vi "SVT UFF58 Write Time Waveform (N Ch).vi"(0 "file refnum":refnum<k20>, 1 "ID lines (1-3)":T2[](array[typedef]), 2 "data precision (double-precision:1)":T1=1 items=["single-precision", "double-precision"], 5 "waveforms":waveform(dbl)[](array[waveform]), 11 "error in (no error)":errorcluster) -> (4 "dup file refnum":refnum<k20>, 6 "function refnums":refnum<k20>[](array[refnum]), 15 "error out":errorcluster)   [LabVIEW 2017, in "SoundVib_UFF58.lvlib"]
doc: "Writes data to the UFF58 (universal file format) file specified by the <B>file refnum</B> input. This VI also writes the fields in records 1, 2, and 3, <B>ID lines (1-3)</B>. You can write a single time domain waveform, multiple time domain waveforms, a single real frequency spectrum, multiple real frequency spectra, a single complex frequency spectrum, multiple complex frequency spectra, or generic data to a UFF file. If a frequency spectrum is in decibels, this VI converts the spectrum to linear before writing to the UFF58 file. The default instance, SVT UFF58 Write Time Waveform (1 Ch), writes a single time domain waveform to the file specified by the <B>file refnum</B> input. Wire data to the <B>file refnum</B> input to determine the polymorphic instance to use or manually select the instance."
uses:
  <vilib>/addons/Sound and Vibration/svt_UFF58/SoundVib_UFF58.lvlib
  <vilib>/addons/Sound and Vibration/svt_UFF58/subVIs/sv_IDLines123.ctl
  <vilib>/addons/Sound and Vibration/svt_UFF58/subVIs/sv_UFF58 Data Precision.ctl
  <vilib>/addons/Sound and Vibration/svt_UFF58/subVIs/sv_UFF58 Check Data Valid (Time) (NCh).vi
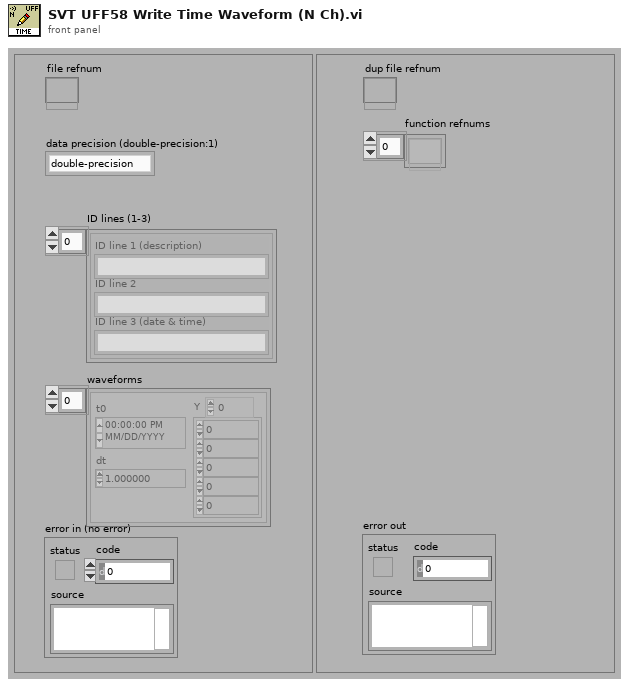
[diagram p1: front panel]
types:
  T1 = typedef "SoundVib_UFF58.lvlib/sv_UFF58 Data Precision.ctl" = u32
  T2 = typedef "SoundVib_UFF58.lvlib/sv_IDLines123.ctl" = cluster{"ID line 1 (description)":string, "ID line 2":string, "ID line 3 (date & time)":string}
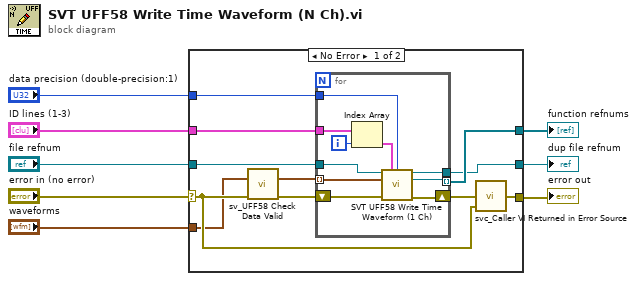
[diagram p0: block diagram]
diagram:
  n1 = case shown="No Error" "error in (no error)" {
    selector: "error in (no error)" -> [w12 w30]
    tunnel: "file refnum" -> [w19 w31]
    tunnel: "ID lines (1-3)" -> [w10 _]
    tunnel: "waveforms" -> [w11 _]
    tunnel: [w18 _] -> w5
    tunnel: [w13 w30] -> w4
    tunnel: [w17 w31] -> w3
    tunnel: "data precision (double-precision:1)" -> [w9 _]
    frame No Error {
      n2 = call-poly <vilib>:"sv_UFF58 Check Data Valid.vi"("waveforms"=w11, "error in (no error)"=w12) -> ("dup waveforms"=w16:waveform(dbl)[], "error out"=w15:errorcluster)  [unwired: 12 in]
      n3 = for {
        shift-right: [w27] -> w14
        shift-left: w15 -> [w28]
        tunnel: w19 -> [w29]
        tunnel: w10 -> [w24]
        tunnel: [w26] -> w17
        tunnel: [w25] -> w18 mode=indexing
        tunnel: w16 -> [w22] mode=indexing
        tunnel: w9 -> [w20]
        i -> [w23]
        n4 = Index Array(array=w24, index=w23) -> (element=w21:T2)
        n5 = call <vilib>:"SVT UFF58 Write Time Waveform (1 Ch).vi"("file refnum"=w29, "ID lines (1-3)"=w21, "data precision (double-precision:1)"=w20, "waveform"=w22, "error in (no error)"=w28) -> ("dup file refnum"=w26:refnum<k20>, "function refnum"=w25:refnum<k20>, "error out"=w27:errorcluster)  [unwired: 8 in]
      }
      n6 = call <vilib>:"svc_Caller VI Returned in Error Source.vi"("warning input to caller"=w12, "error in (no error)"=w14) -> ("error out"=w13:errorcluster)  [unwired: 3 in]
    }
    frame Error {
    }
  }
  "function refnums" <- w5
  "dup file refnum" <- w3
  "error out" <- w4
